vi "Atto DRY Interface download Sample Temperature Sensor Calibration Curve.vi"(8 "error in (no error)":errorcluster, 11 "SavePath":string) -> (0 "error out":errorcluster, 2 "function return":i32, 3 "SavePath out":string)   [LabVIEW 2016, in "attoDRYLib.lvlib"]
doc: "int32_t __cdecl AttoDRY_Interface_downloadSampleTemperatureSensorCalibrationCurve(\n char SavePath[]);"
uses:
  <userlib>/attoDRYLib/attoDRYLib.lvlib
  <userlib>/attoDRYLib/attoDRYLib.dll
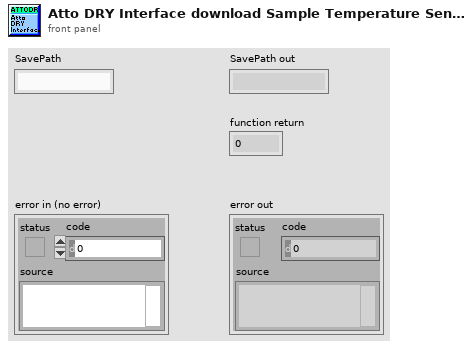
[diagram p1: front panel]
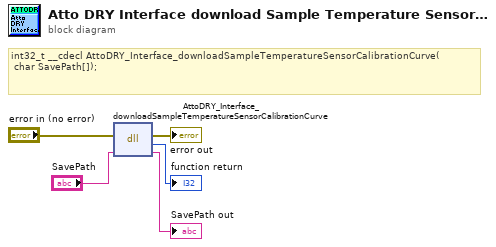
[diagram p0: block diagram]
diagram:
  # "int32_t __cdecl AttoDRY_Interface_downloadSampleTemperatureSensorCalibrationCurve(\n\tchar SavePath[]);"
  n1 = dll-call lib="C:/Program Files (x86)/National Instruments/LabVIEW 2016/user.lib/attoDRYLib/attoDRYLib.*" fn="AttoDRY_Interface_downloadSampleTemperatureSensorCalibrationCurve"(error in="error in (no error)", "SavePath"="SavePath") -> (error out=→"error out":errorcluster, →"function return":i32, "SavePath"=→"SavePath out":string)  [unwired: 2 in, 1 out]
